vi "Read Independent Variables.vi"(8 "error in (no error)":errorcluster, 11 "Scanner.lvclass in":refnum<class "Scanner.lvclass">) -> (0 "error out":errorcluster, 1 "size":i32, 2 "Independent Variables":dbl[](array[numeric]), 3 "Scanner.lvclass out":refnum<class "Scanner.lvclass">, 4 "min value":dbl, 5 "max value":dbl)   [LabVIEW 2009, in "Scanner.lvclass"]
doc: "Return the internal array of independent variables for this Scanner, e.g., to write out to a file. Use this method with extreme caution, since it breaks the encapsulation for this class. Do not use it to manipulate a Scanner's internal state."
uses:
  Scanner.lvclass
  Scanner.lvclass/Scanner.ctl
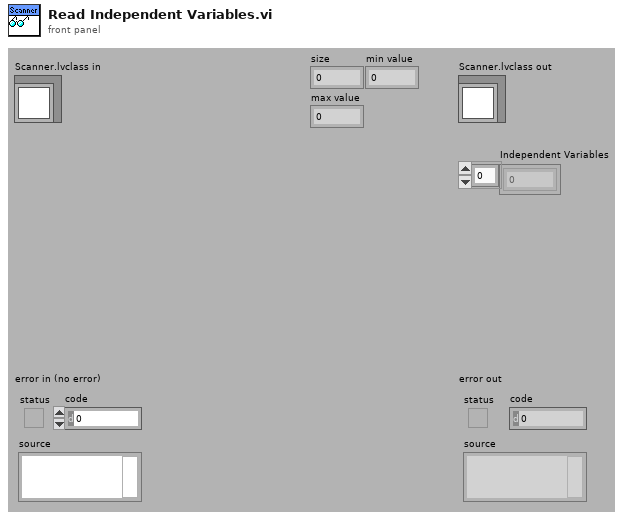
[diagram p1: front panel]
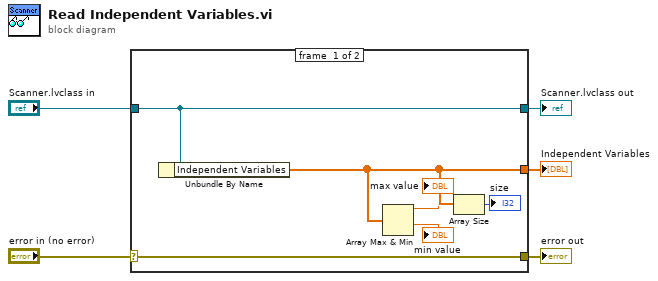
[diagram p0: block diagram]
diagram:
  n1 = case shown="No Error" "error in (no error)" {
    selector: "error in (no error)" -> [w11 w12]
    tunnel: [w11 w12] -> w4
    tunnel: [w10 w13] -> w2
    tunnel: "Scanner.lvclass in" -> [w10 w13]
    tunnel: [w8 _] -> w1
    frame #0 {
      n2 = Unbundle By Name(w10) -> ("Independent Variables"=w8:dbl[])
      n3 = Array Max & Min(array=w8) -> (max value=→"max value":dbl, min value=→"min value":dbl)  [unwired: 2 out]
      n4 = Array Size(array=w8) -> (size(s)=→"size":i32)
    }
    frame #1 {
    }
  }
  "error out" <- w4
  "Scanner.lvclass out" <- w2
  "Independent Variables" <- w1
